vi "gentec-M-Link.Set Single Shot Energy.vi"(0 "VISA resource In":refnum<visa-resource-name>, 2 "Enable Single Shot Energy":bool, 5 "error in (no error)":errorcluster) -> (11 "Data Read":string, 13 "Read Timeout":bool, 14 "VISA resource Out":refnum<visa-resource-name>, 16 "Success":bool, 17 "no Thermopyle Head":bool, 19 "error out":errorcluster)   [LabVIEW 2014, in "gentec-M-Link - Driver.lvlib"]
doc: "Data to write: sse0 or sse1\n\nCommand only. Enables (true) or disables (false) Single Shot Energy (SSE) for Thermopile Heads. If such a head is not in use, it replies \"Thermopile Head Only\", otherwise \"ok\"."
uses:
  gentec-M-Link - Driver.lvlib
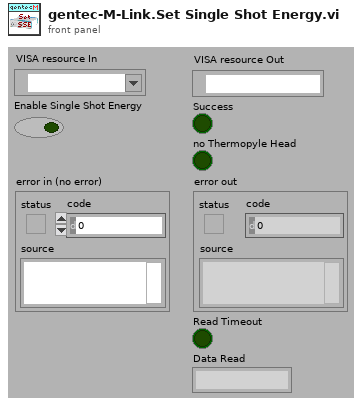
[diagram p1: front panel]
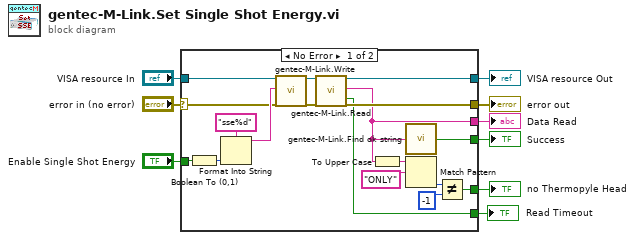
[diagram p0: block diagram]
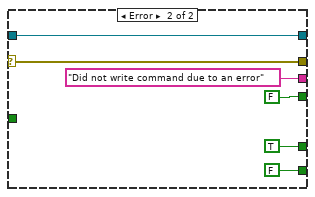
[diagram p2: hidden frame]
diagram:
  n1 = case shown="No Error" "error in (no error)" {
    selector: "error in (no error)" -> [w24 w33]
    tunnel: [w26 w33] -> w8
    tunnel: "VISA resource In" -> [w23 w32]
    tunnel: [w20 FALSE ("Found")] -> w6
    tunnel: [w19 w32] -> w5
    tunnel: "Enable Single Shot Energy" -> [w18 _]
    tunnel: [w16 "Did not write command due to an error" ("Data Read")] -> w3
    tunnel: [w11 TRUE] -> w2
    tunnel: [w10 FALSE ("Read Timeout")] -> w1
    frame No Error {
      n2 = Boolean To (0,1)(Boolean=w18) -> (0, 1=w17:i16)
      n3 = Format Into String(format string="sse%d", w17) -> (resulting string=w25:string)  [unwired: 2 in, 1 out]
      n4 = call "gentec-M-Link.Write.vi"("VISA resource (In)"=w23, "Data To Write"=w25, "error in (no error)"=w24) -> ("VISA resource (Out)"=w22:refnum<visa-resource-name>, "error out"=w21:errorcluster)  [unwired: 14 in, 1 out]
      n5 = call "gentec-M-Link.Read.vi"("VISA resource (In)"=w22, "error in (no error)"=w21) -> ("VISA resource (Out)"=w19:refnum<visa-resource-name>, "Data Read"=w16:string, "Read Timeout"=w10:bool, "error out"=w26:errorcluster)  [unwired: 13 in, 1 out]
      n6 = To Upper Case(1:w16) -> (0:w15:string)
      n7 = call "gentec-M-Link.Find ok string.vi"("string"=w16) -> ("Found"=w20:bool)
      n8 = Match Pattern(string=w15, regular expression="ONLY") -> (offset past match=w13:i32)  [unwired: 1 in, 3 out]
      n9 = Not Equal?(x=w13, y=-1) -> (x != y?=w11:bool)
    }
    frame Error {
    }
  }
  "error out" <- w8
  "Success" <- w6
  "VISA resource Out" <- w5
  "Data Read" <- w3
  "no Thermopyle Head" <- w2
  "Read Timeout" <- w1
